vi "FPGA open.vi"(8 "error in":errorcluster) -> (0 "error out":errorcluster)   [LabVIEW 2019, in "my FPGA lib.lvlib"]
uses:
  my FPGA lib.lvlib
  <vilib>/FPGAPlugInAG/myRIO-1900/niLvFpga_Open_myRIO-1900.vi
  <vilib>/rvi/interface/common/dynamic/niFpgaDynamicAddResources.vi
  <vilib>/rvi/interface/nirviOpenFPGA/nirviOpenFPGA.xnode
  tankfpga_FPGATarget_FPGA-test001_q+SCbNOC5hc.lvbitx
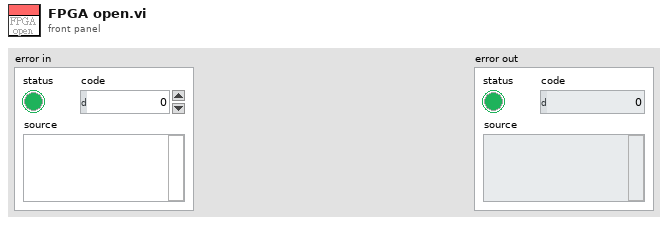
[diagram p1: front panel]
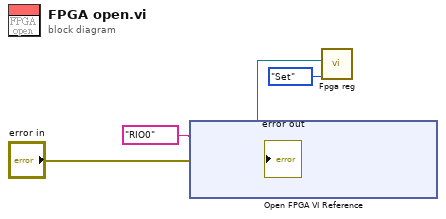
[diagram p0: block diagram]
diagram:
  n1 = xnode "Open FPGA VI Reference"("error in"="error in", "resource name"=tag "RIO0") -> ("FPGA VI Reference Out"=w5:refnum<k20>, "error out"=→"error out":errorcluster)
  n2 = call "Fpga reg.vi"("Mode"=enum16{"Get", "Set"}."Set", "FPGA VI Reference Set"=w5) -> ()  [unwired: 9 in, 1 out]
